vi "receive_00archived.vi"() -> ()   [LabVIEW 2015]
uses:
  <instrlib>/niUSRP/niUSRP Fetch Rx Data (CDB Cluster).vi
  <vilib>/addons/Modulation/Analog/MT Demodulate AM (DSB).vi
  <vilib>/addons/Modulation/niAMT.lvlib
panel:
  in  "modulation index":dbl=1.0 format="%.2f"
  out "AM demodulated":waveform(dbl)(graph)
  in  "Write to File":bool=TRUE caption="Enable"
  out "output bit stream":i8[](array[numeric])
  in  "active antenna":string="RX1"
  in  "Channels":string(combo)="1"
  out "Waveform Magnitude":cluster{"t0":dbl, "dt":dbl, "Y":dbl[]}(graph)
  in  "Stop":bool
  out "coerced gain":dbl format="%#_6f"
  out "coerced carrier frequency":dbl=100000.0 format="%#_6p"
  out "coerced IQ rate":dbl=100000.0 format="%#_6p"
  in  "gain":dbl format="%#_6f"
  in  "carrier frequency":dbl=100000.0 format="%#_6p"
  in  "IQ rate":dbl=100000.0 format="%#_6p"
  in  "number of samples":i64=100000
  in  "timeout":dbl=10.0
  out "error out":errorcluster
  in  "device names":refnum<k15>
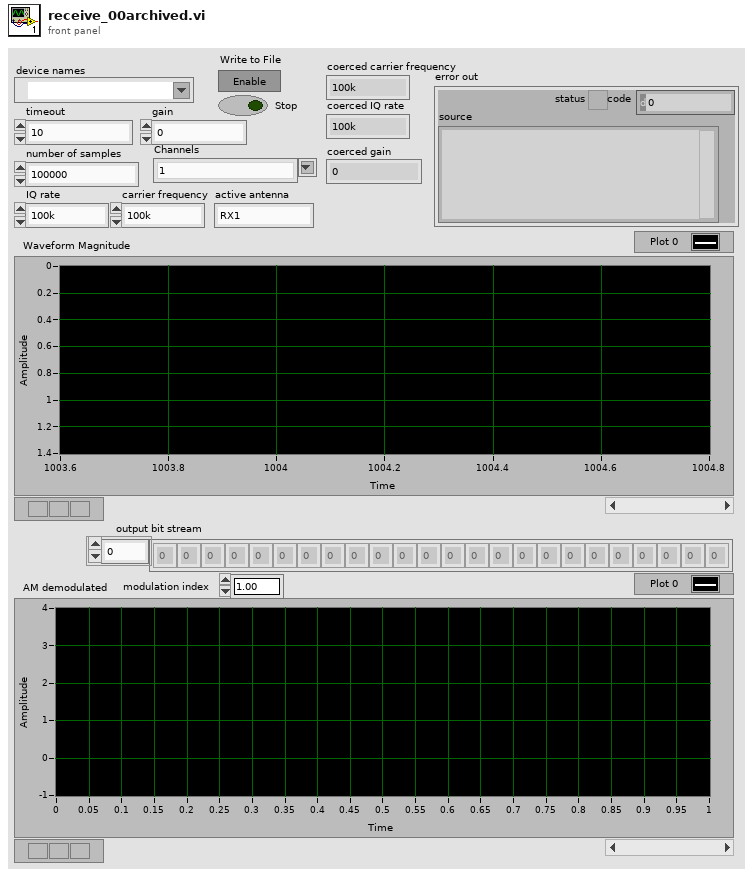
[diagram p1: front panel]
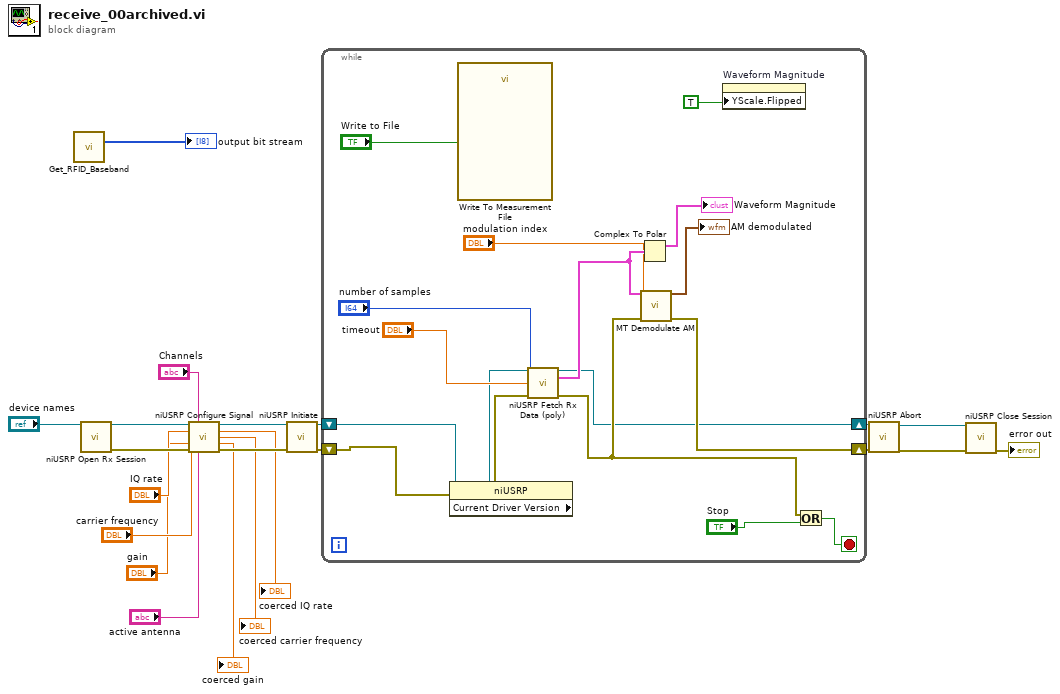
[diagram p0: block diagram]
diagram:
  n1 = call "Get_RFID_Baseband.vi"() -> ("output bit stream"=→"output bit stream":i8[])  [unwired: 14 in, 1 out]
  n2 = call <instrlib>:"niUSRP Open Rx Session.vi"("device names"="device names") -> ("session handle out"=w20:refnum<k15>, "error out"=w19:errorcluster)  [unwired: 13 in]
  n3 = call <instrlib>:"niUSRP Configure Signal.vi"("session handle"=w20, "channel list"="Channels", "IQ rate"="IQ rate", "carrier frequency"="carrier frequency", "gain"="gain", "error in (no error)"=w19, "active antenna"="active antenna") -> ("session handle out"=w18:refnum<k15>, "coerced IQ rate"=→"coerced IQ rate":dbl, "coerced carrier frequency"=→"coerced carrier frequency":dbl, "coerced gain"=→"coerced gain":dbl, "error out"=w17:errorcluster)  [unwired: 4 in]
  n4 = call <instrlib>:"niUSRP Initiate.vi"("session handle"=w18, "error in (no error)"=w17) -> ("session handle out"=w16:refnum<k15>, "error out"=w15:errorcluster)  [unwired: 12 in]
  n5 = while {
    shift-right: [w26] -> w14
    shift-left: w16 -> [w25]
    shift-right: [w30] -> w13
    shift-left: w15 -> [w23]
    stop <- w36 stop-if-true
    n6 = property on="Property Node" class="niUSRP" props=["Current Driver Version"](reference=w25, error in=w23) -> (reference out=w24:refnum<k15>, error out=w22:errorcluster)  [unwired: 1 out]
    n7 = call "Write To Measurement File"("Enable"="Write to File") -> ()  [unwired: 16 in, 3 out]
    n8 = call-poly <instrlib>:"niUSRP Fetch Rx Data (poly).vi"("session handle"=w24, "number of samples"="number of samples", "timeout"="timeout", "error in (no error)"=w22) -> ("session handle out"=w26:refnum<k15>, "data"=w32:cluster{"t0":dbl, "dt":dbl, "Y":cdb[]}, "error out"=w31:errorcluster)  [unwired: 8 in, 1 out]
    n9 = Complex To Polar(r * e^(i*theta)=w32) -> (r=→"Waveform Magnitude":cluster{"t0":dbl, "dt":dbl, "Y":dbl[]})  [unwired: 1 out]
    n10 = call-poly <vilib>:"MT Demodulate AM.vi"("AM modulated waveform"=w32, "modulation index"="modulation index", "error in (no error)"=w31) -> ("AM demodulated waveform"=→"AM demodulated":waveform(dbl), "error out"=w30:errorcluster)  [unwired: 10 in, 1 out]
    n11 = property on="Waveform Magnitude" class="WFGraph (strict)"("YScale.Flipped"=TRUE ("Y Scale.Flipped")) -> ()  [unwired: 2 in, 2 out]
    n12 = Or(x=w31, y="Stop") -> (x .or. y?=w36:bool)
  }
  n13 = call <instrlib>:"niUSRP Abort.vi"("session handle"=w14, "error in (no error)"=w13) -> ("session handle out"=w12:refnum<k15>, "error out"=w11:errorcluster)  [unwired: 12 in]
  n14 = call <instrlib>:"niUSRP Close Session.vi"("session handle"=w12, "error in (no error)"=w11) -> ("error out"=→"error out":errorcluster)  [unwired: 13 in]
